vi "Run.vi"(8 "error in (no error)":errorcluster, 10 "OTP Cluster Out":T1, 11 "LCR-Measurement in":refnum<class "OTP_LCR_Meas.lvclass">) -> (0 "error out":errorcluster, 1 "Parameters":cluster{"Name":string, "Value":string}[](array[cluster]), 2 "Canceled":bool, 3 "LCR-Measurement out":refnum<class "OTP_LCR_Meas.lvclass">)   [LabVIEW 2020, in "OTP_LCR_Meas.lvclass"]
doc: "This is the main test vi. It is here that the test is implemented."
uses:
  OTP_LCR_Meas.lvclass
  C:/Sandbox/Git_Sandbox/WiSpry Test Framework source code (LV20)/WiSpry Test Framework/Measurements/Measurement.lvclass
  Controls/OTP_Cluster.ctl
  Controls/Run States.ctl
  Instruments/LCR Meter/Controls/Function.ctl
  Devices/Controls/Change setting mode enum.ctl
  Measurement.lvclass/Measurement.ctl
  XML Handler/Controls/Result Cluster.ctl
  Support VI/Update parameters (single).vi
  Support VI/Update parameters (array).vi
  Measurement.lvclass
  Instruments/LCR Meter/LCR Meter.lvclass
  Devices/Device.lvclass
  Devices/PIC-device/PIC-Device.lvclass
  XML Handler/XML Handler.lvclass
  Instruments/Power Supply/Power Supply.lvclass
  Instruments/Digital Multimeter/Digital Multimeter.lvclass
panel:
  out "Tab Control":enum32{"Page 1", "Page 2"}(tab)
  out "XY Graph":T2(graph)
  out "Waveform Chart":dbl[](graph)
  in  "Cancel Button":bool
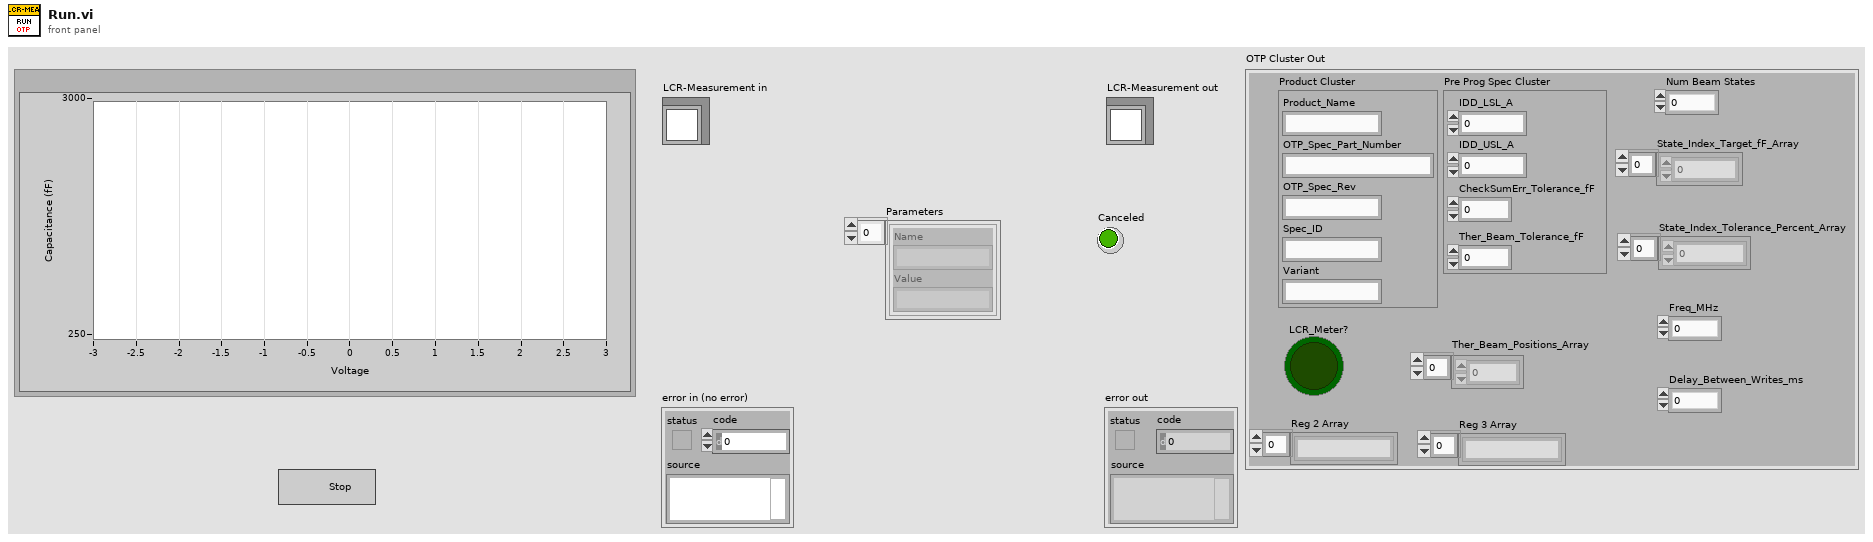
[diagram p1: front panel]
types:
  T1 = typedef "OTP_Cluster.ctl" = cluster{"Product Cluster":cluster{"Product_Name":string, "OTP_Spec_Part_Number":string, "OTP_Spec_Rev":string, "Spec_ID":string, "Variant":string}, "Pre Prog Spec Cluster":cluster{"IDD_LSL_A":dbl, "IDD_USL_A":dbl, "CheckSumErr_Tolerance_fF":dbl, "Ther_Beam_Tolerance_fF":dbl}, "LCR_Meter?":bool, "Reg 2 Array":string[], "Reg 3 Array":string[], "Num Beam States":i32, "State_Index_Target_fF_Array":dbl[], "State_Index_Tolerance_Percent_Array":dbl[], "Freq_MHz":dbl, "Delay_Between_Writes_ms":i32, "Ther_Beam_Positions_Array":i8[]}
  T2 = cluster{"Bias Voltages (V)":dbl[], "Capacitances (fF)":dbl[]}[]
  T3 = typedef "Measurement.lvclass/Run States.ctl" = enum16{"Init", "Set Device", "Read Environment", "Measure", "Done"}
  T4 = cluster{"Bias Voltages (V)":dbl[], "Capacitances (fF)":dbl[]}
  T5 = typedef "LCR Meter.lvclass/Function.ctl" = enum16{"Cp-D", "Cp-Q", "Cp-G", "Cp-Rp", "Cs-D", "Cs-Q", "Cs-Rs", "Lp-D", "Lp-Q", "Lp-G", "Lp-Rp", "Lp-Rdc", "Ls-D", "Ls-Q", "Ls-Rs", "Ls-Rdc", "R-X", "Z-thd", "Z-thr", "G-B", "Y-thd", "Y-thr", "Vdc-Idc"}
  T6 = typedef "PIC-Device.lvclass/Change setting mode enum.ctl" = enum16{"Init", "Next", "Reset"}
  T7 = typedef "XML Handler.lvclass/Result Cluster.ctl" = cluster{"Name":string, "Value":string}
  T8 = cluster{"Value":string, "Capacitance (fF)":string}
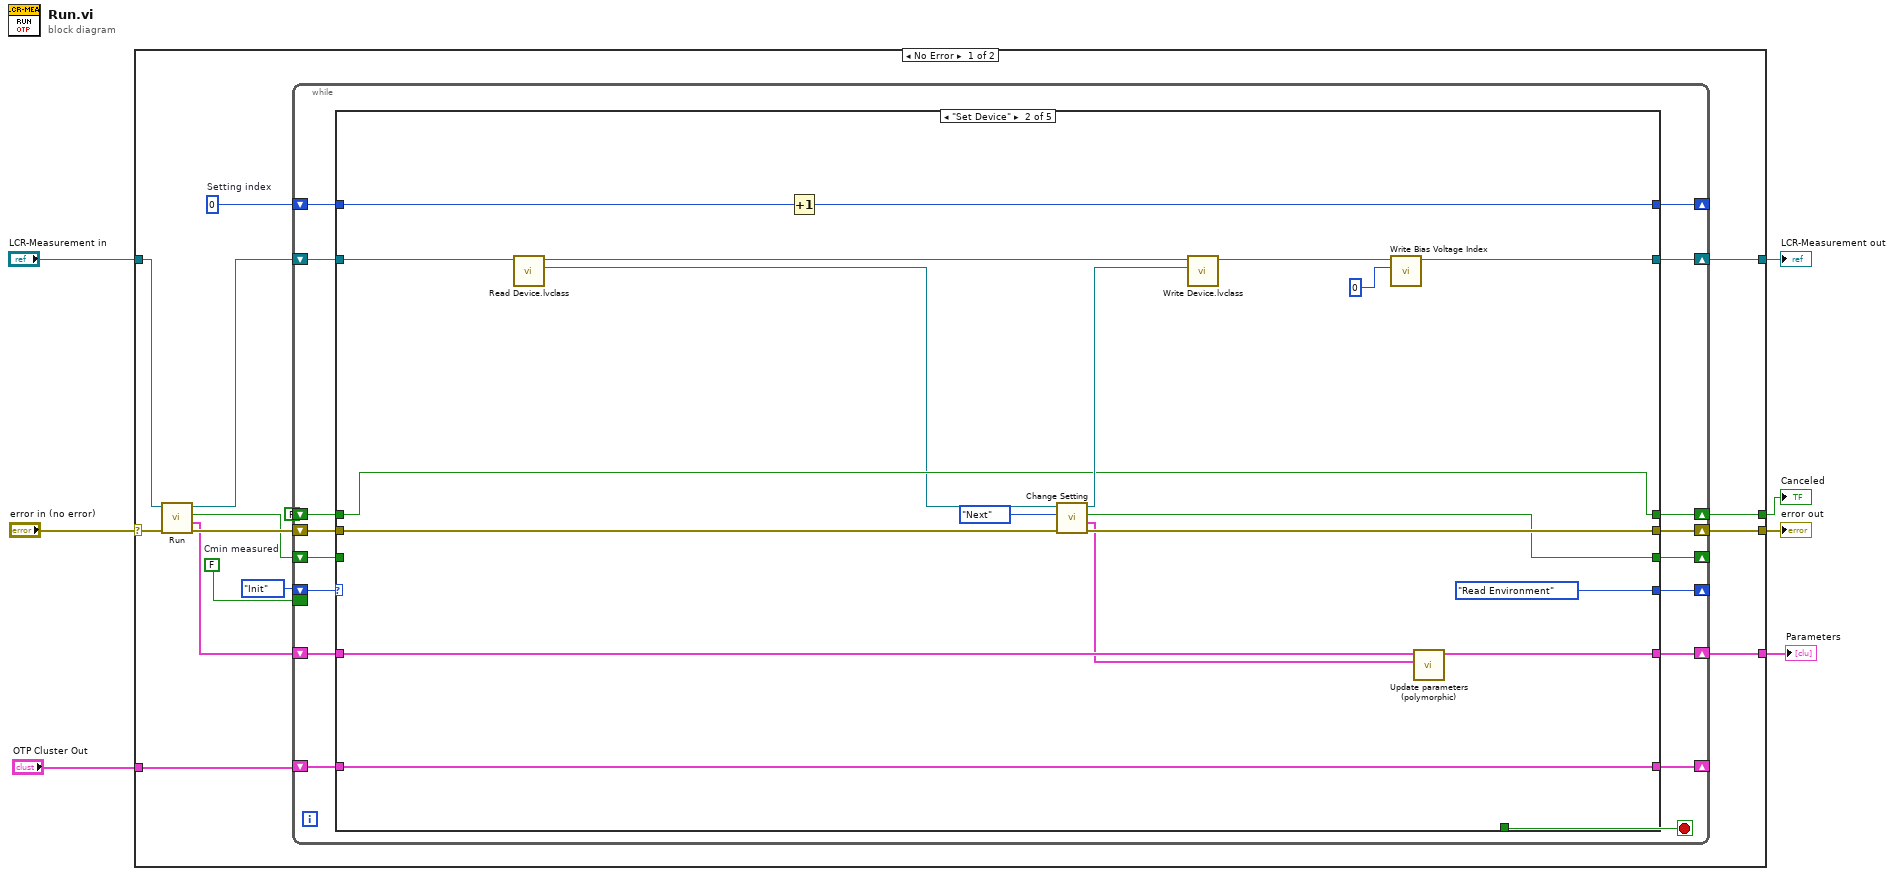
[diagram p0: block diagram]
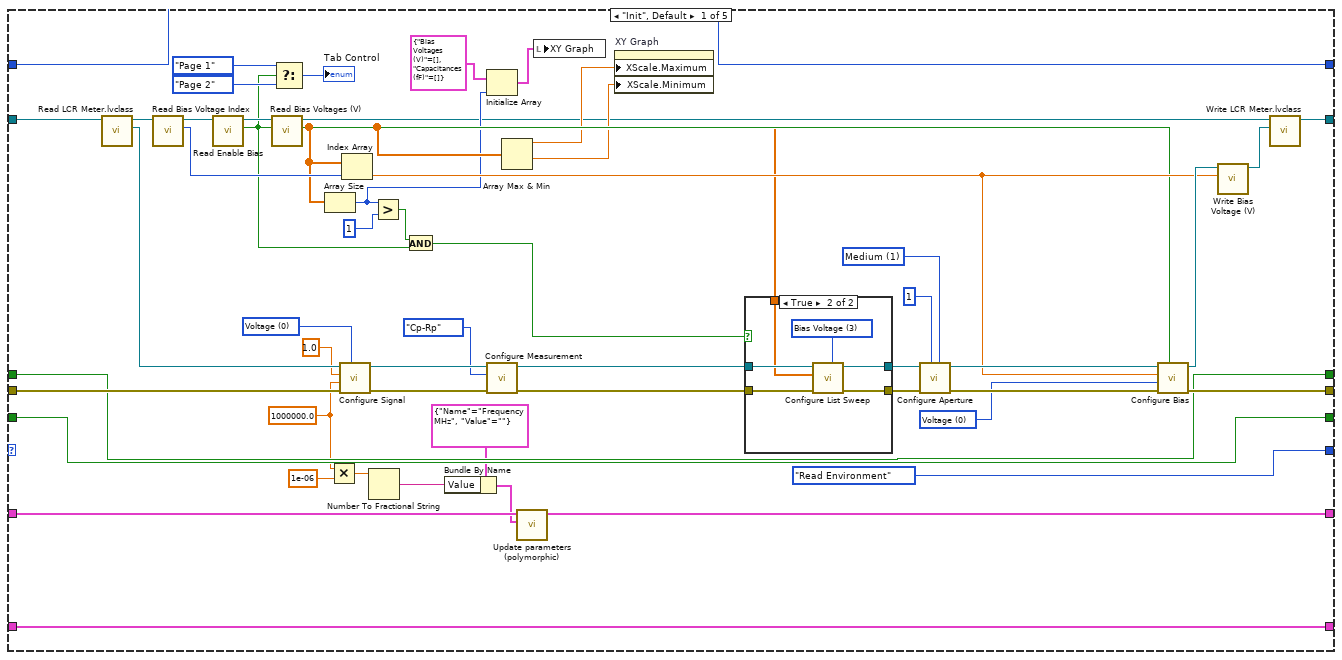
[diagram p2: hidden frame]
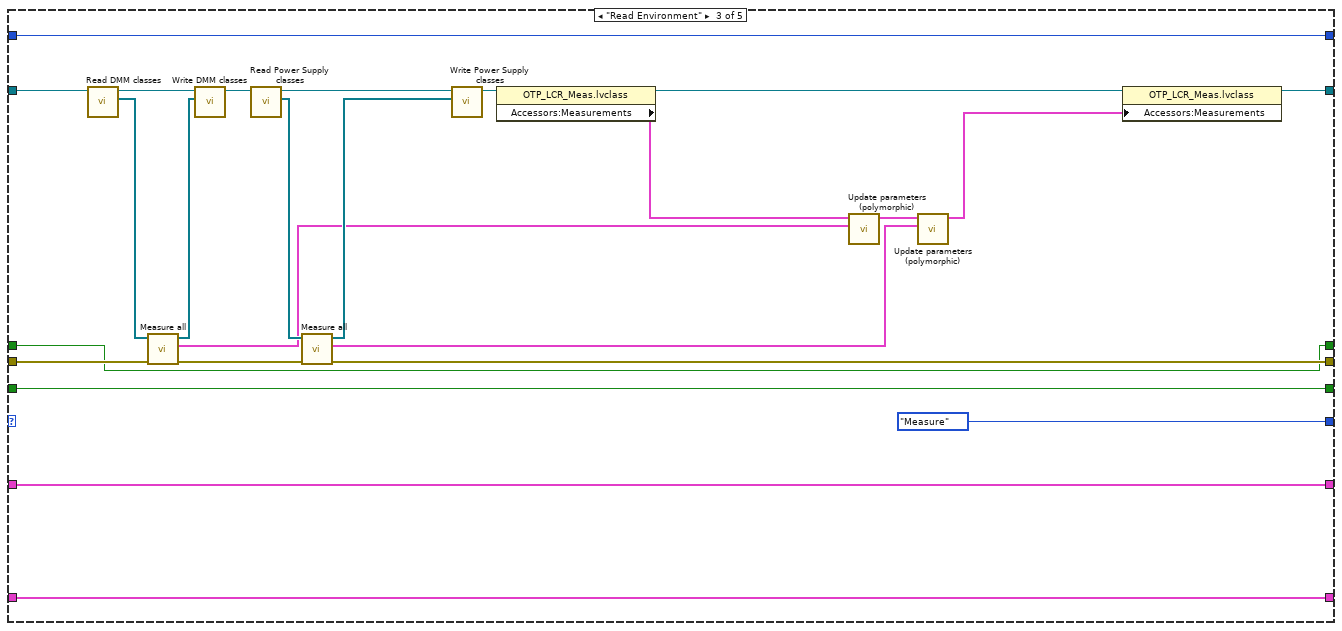
[diagram p4: hidden frame]
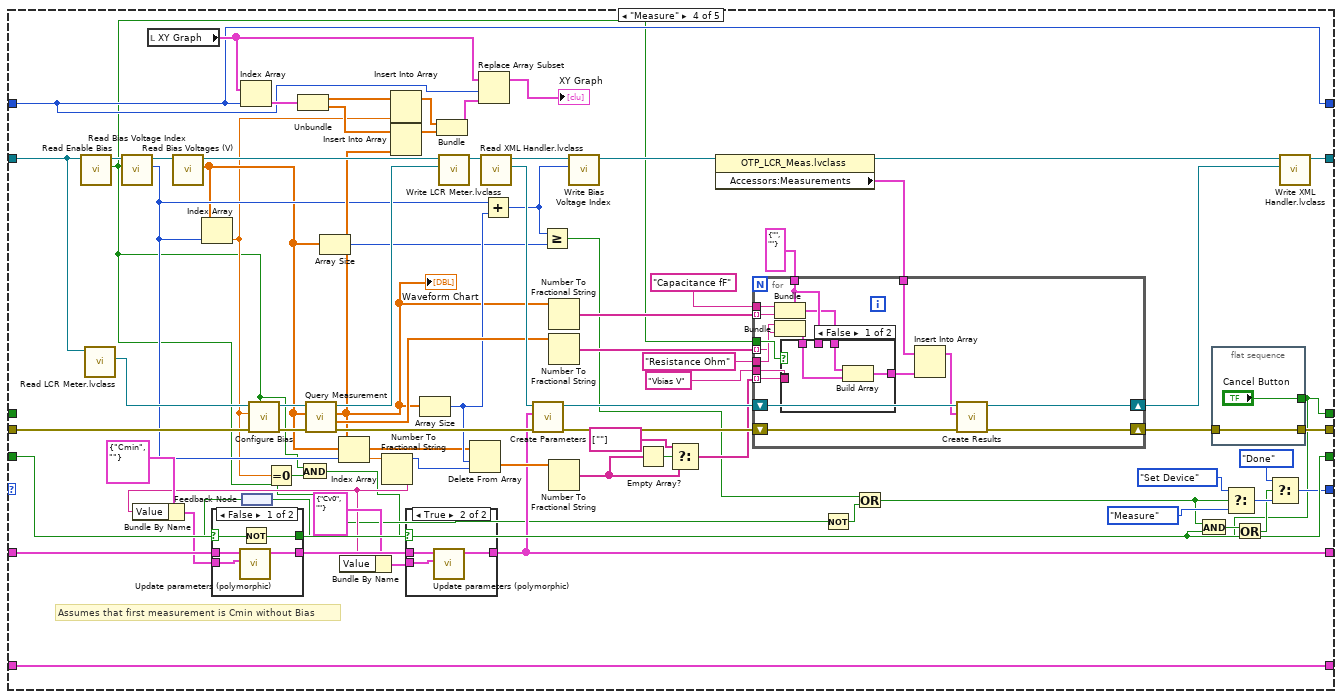
[diagram p5: hidden frame]
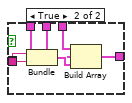
[diagram p8: hidden frame]
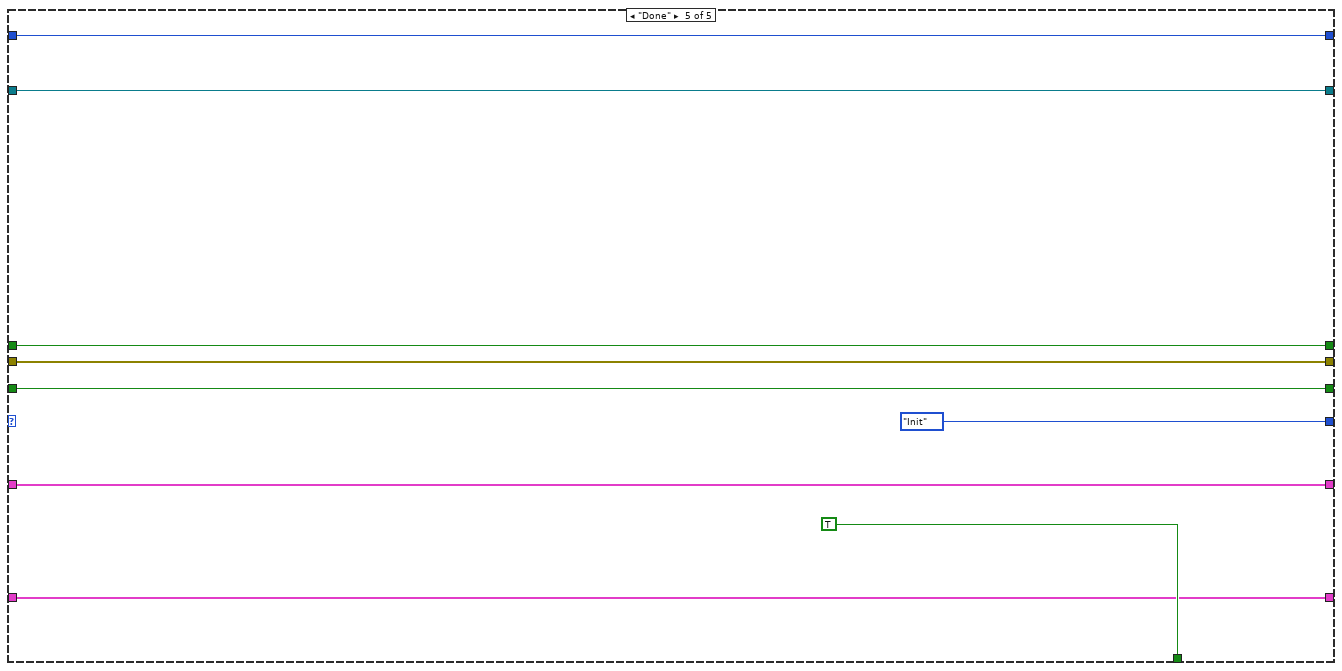
[diagram p9: hidden frame]
diagram:
  n1 = case shown="No Error" "error in (no error)" {
    selector: "error in (no error)" -> [w22 w272]
    tunnel: "LCR-Measurement in" -> [w21 w271]
    tunnel: [w19 w272] -> w6
    tunnel: [w17 w271] -> w5
    tunnel: [w16 _] -> w4
    tunnel: [w15 _] -> w3
    tunnel: "OTP Cluster Out" -> [w8 _]
    frame No Error {
      w10 = 0  # Setting index
      w11 = FALSE  # Cmin measured
      n2 = call-parent "Run.vi"("error in (no error)"=w22, "Measurements in"=w21) -> ("error out"=w20:errorcluster, "Parameters"=w12:cluster{"Name":string, "Value":string}[], "Canceled"=w14:bool, "Measurements out"=w18:refnum<class "OTP_LCR_Meas.lvclass">)  [unwired: 6 in]
      n3 = while {
        shift-right: [w38] -> w19
        shift-left: w20 -> [w39]
        shift-right: [w37] -> w17
        shift-left: w18 -> [w36]
        shift-right: [w34] -> _
        shift-left: Run_States."Init" ("Run states") -> [w25]
        shift-right: [w32] -> w15
        shift-left: w12 -> [w33]
        shift-right: [w31] -> _
        shift-left: w14 -> [w30]
        shift-right: [w28] -> w16
        shift-left: FALSE ("Cancel Button") -> [w29]
        border: w11 -> [_]
        shift-right: [w26] -> _
        shift-left: w10 -> [w27]
        shift-right: [w23] -> _
        shift-left: w8 -> [w24]
        stop <- w35 stop-if-true
        n4 = case shown="\"Set Device\"" w25 {
          tunnel: w39 -> [w84 w118 w136 w194 w270]
          tunnel: [w83 w117 w132 w183 w270] -> w38
          tunnel: [w81 w108 w127 w214 w269] -> w37
          tunnel: w36 -> [w82 w103 w143 w200 w269]
          tunnel: [_ _ _ _ TRUE] -> w35
          tunnel: [Run_States."Read Environment" ("Run states") Run_States."Read Environment" ("Run states") Run_States."Measure" ("Run states") w217 Run_States."Init" ("Run states")] -> w34
          tunnel: [w57 w109 w128 w181 w264] -> w28
          tunnel: w33 -> [w56 w114 w126 w177 w265]
          tunnel: [w55 w112 w126 w154 w265] -> w32
          tunnel: [w58 w110 w142 w219 w266] -> w31
          tunnel: w30 -> [w58 _ w142 w219 w266]
          tunnel: w29 -> [w57 w109 w128 _ w264]
          tunnel: w27 -> [w42 w105 w121 w162 w263]
          tunnel: [w42 w104 w121 w162 w263] -> w26
          tunnel: w24 -> [w40 w102 w120 w145 w262]
          tunnel: [w40 w102 w120 w145 w262] -> w23
          frame "Init", Default {
            w67 = u16 0 items=["Voltage", "Current"] ("DC Bias Type (0: Voltage)")
            w75 = u16 1 items=["Short", "Medium", "Long"] ("Measurement Time (1: Medium)")
            w53 = 1000000.0 ("Signal Frequency (1000 Hz)")
            w79 = u16 0 items=["Voltage", "Current"] ("Signal Type (0: Voltage)")
            n5 = call-dynamic "Read LCR Meter.lvclass.vi"("LCR-Measurement in"=w82) -> ("LCR Meter.lvclass"=w80:refnum<class "LCR Meter.lvclass">, "LCR-Measurement out"=w71:refnum<class "OTP_LCR_Meas.lvclass">)  [unwired: 9 in]
            n6 = call-dynamic "Read Bias Voltage Index.vi"("LCR-Measurement in"=w71) -> ("Bias Voltage Index"=w69:i32, "LCR-Measurement out"=w70:refnum<class "OTP_LCR_Meas.lvclass">)  [unwired: 9 in]
            n7 = call-dynamic "Read Enable Bias.vi"("LCR-Measurement in"=w70) -> ("Enable Bias"=w60:bool, "LCR-Measurement out"=w72:refnum<class "OTP_LCR_Meas.lvclass">)  [unwired: 9 in]
            n8 = call-dynamic "Read Bias Voltages (V).vi"("LCR-Measurement in"=w72) -> ("Bias Voltages (V)"=w48:dbl[], "LCR-Measurement out"=w41:refnum<class "OTP_LCR_Meas.lvclass">)  [unwired: 9 in]
            n9 = Select(t=enum32{"Page 1", "Page 2"}."Page 1" ("Tab Control"), s=w60, f=enum32{"Page 1", "Page 2"}."Page 2" ("Tab Control")) -> (s? t:f=→"Tab Control":enum32{"Page 1", "Page 2"})
            n10 = Array Size(array=w48) -> (size(s)=w44:i32)
            n11 = Multiply(x=w53, y=1e-06) -> (x*y=w51:dbl)
            n12 = call-dynamic "Configure Signal.vi"("Signal Type (0: Voltage)"=w79, "error in (no error)"=w84, "Signal Frequency (1 MHz)"=w53, "Signal Level (1.0 V)"=1.0, "LCR Meter in"=w80) -> ("error out"=w91:errorcluster, "LCR Meter out"=w92:refnum<class "LCR Meter.lvclass">)  [unwired: 5 in]
            n13 = Index Array(array=w48, index=w69) -> (element=w68:dbl)
            n14 = Number To Fractional String(number=w51) -> (F-format string=w50:string)  [unwired: 3 in]
            n15 = Greater?(x=w44, y=1) -> (0:w64:bool)
            n16 = And(x=w64, y=w60) -> (x .and. y?=w66:bool)
            n17 = Bundle By Name(cluster=cluster{"Name":string, "Value":string} {"Name"="Frequency MHz", "Value"=""} ("New Parameter"), "Value"=w50) -> (w49:cluster{"Name":string, "Value":string})
            n18 = Initialize Array(T4 {"Bias Voltages (V)"=[], "Capacitances (fF)"=[]} ("XY Graph"), w44) -> (w43:T2)
            n19 = call-dynamic "Configure Measurement.vi"("error in (no error)"=w91, "Function (0: Cp-D)"=Function."Cp-Rp", "LCR Meter in"=w92) -> ("error out"=w89:errorcluster, "LCR Meter out"=w90:refnum<class "LCR Meter.lvclass">)  [unwired: 7 in]
            n20 = Array Max & Min(array=w48) -> (max value=w47:dbl, min value=w46:dbl)  [unwired: 2 out]
            n21 = call-poly "Update parameters (polymorphic).vi"("New Parameter"=w49, "Parameters"=w56) -> ("Parameters Out"=w55:cluster{"Name":string, "Value":string}[])  [unwired: 9 in]
            n22 = local write "XY Graph"(w43) -> ()
            n23 = property on="XY Graph" class="XYGraph (strict)"("XScale.Maximum"=w47, "XScale.Minimum"=w46) -> ()  [unwired: 2 in, 2 out]
            n24 = case shown="True" w66 {
              tunnel: w90 -> [w94 w100]
              tunnel: w89 -> [w93 w99]
              tunnel: [w94 w98] -> w88
              tunnel: [w93 w97] -> w87
              tunnel: w48 -> [_ w96]
              frame False {
              }
              frame True {
                w95 = u16 3 items=["Frequency", "Voltage", "Current", "Bias Voltage", "Bias Current", "DC Source Voltage"] ("Sweep Function A (0: Frequency)")
                n25 = call-dynamic "Configure List Sweep.vi"("Sweep Function A (0: Frequency)"=w95, "error in (no error)"=w99, "Sweep Point Array"=w96, "LCR Meter in"=w100) -> ("error out"=w97:errorcluster, "LCR Meter out"=w98:refnum<class "LCR Meter.lvclass">)  [unwired: 6 in]
              }
            }
            n26 = call-dynamic "Configure Aperture.vi"("Measurement Time (1: Medium)"=w75, "Averaging Factor (1)"=1, "error in (no error)"=w87, "LCR Meter in"=w88) -> ("error out"=w85:errorcluster, "LCR Meter out"=w86:refnum<class "LCR Meter.lvclass">)  [unwired: 6 in]
            n27 = call-dynamic "Configure Bias.vi"("DC Bias State (F:Disable)"=w60, "error in (no error)"=w85, "DC Bias Type (0: Voltage)"=w67, "DC Bias Level (0.0 V)"=w68, "LCR Meter in"=w86) -> ("error out"=w83:errorcluster, "LCR Meter out"=w73:refnum<class "LCR Meter.lvclass">)  [unwired: 5 in]
            n28 = call-dynamic "Write Bias Voltage (V).vi"("Bias Voltage (V)"=w68, "LCR Meter in"=w73) -> ("LCR Meter out"=w74:refnum<class "LCR Meter.lvclass">)  [unwired: 9 in]
            n29 = call-dynamic "Write LCR Meter.lvclass.vi"("LCR Meter.lvclass"=w74, "LCR-Measurement in"=w41) -> ("LCR-Measurement out"=w81:refnum<class "OTP_LCR_Meas.lvclass">)  [unwired: 9 in]
          }
          frame "Set Device" {
            n30 = call "Read Device.lvclass.vi"("Measurements in"=w103) -> ("Device.lvclass"=w101:refnum<class "Device.lvclass">, "Measurements out"=w116:refnum<class "OTP_LCR_Meas.lvclass">)  [unwired: 9 in]
            n31 = Increment(x=w105) -> (x+1=w104:i32)
            n32 = call-dynamic "Change Setting.vi"("error in (no error)"=w118, "Change setting mode"=Change_setting_mode_enum."Next", "Device in"=w101) -> ("error out"=w117:errorcluster, "Changes"=w113:cluster{"Name":string, "Value":string}[], "Last setting"=w110:bool, "Device out"=w115:refnum<class "Device.lvclass">)  [unwired: 5 in]
            n33 = call "Write Device.lvclass.vi"("Device.lvclass"=w115, "Measurements in"=w116) -> ("Measurements out"=w107:refnum<class "OTP_LCR_Meas.lvclass">)  [unwired: 9 in]
            n34 = call-dynamic "Write Bias Voltage Index.vi"("Bias Voltage Index"=0, "LCR-Measurement in"=w107) -> ("LCR-Measurement out"=w108:refnum<class "OTP_LCR_Meas.lvclass">)  [unwired: 9 in]
            n35 = call-poly "Update parameters (polymorphic).vi"("New Parameters"=w113, "Parameters"=w114) -> ("Parameters Out"=w112:cluster{"Name":string, "Value":string}[])  [unwired: 9 in]
          }
          frame "Read Environment" {
            n36 = call-dynamic "Read DMM classes.vi"("Measurements in"=w143) -> ("DMM classes"=w133:refnum<class "Digital Multimeter.lvclass">[], "Measurements out"=w144:refnum<class "OTP_LCR_Meas.lvclass">)  [unwired: 9 in]
            n37 = call "Measure all.vi"("error in (no error)"=w136, "Digital Multimeters in"=w133) -> ("error out"=w135:errorcluster, "Measurements"=w131:T7[], "Digital Multimeters out"=w134:refnum<class "Digital Multimeter.lvclass">[])  [unwired: 5 in, 2 out]
            n38 = call-dynamic "Write DMM classes.vi"("DMM classes"=w134, "Measurements in"=w144) -> ("Measurements out"=w140:refnum<class "OTP_LCR_Meas.lvclass">)  [unwired: 9 in]
            n39 = call-dynamic "Read Power Supply classes.vi"("Measurements in"=w140) -> ("Power Supply classes"=w138:refnum<class "Power Supply.lvclass">[], "Measurements out"=w139:refnum<class "OTP_LCR_Meas.lvclass">)  [unwired: 9 in]
            n40 = call "Measure all.vi"("error in (no error)"=w135, "Power Supplies in"=w138) -> ("error out"=w132:errorcluster, "Measurements"=w129:T7[], "Power Supplies out"=w137:refnum<class "Power Supply.lvclass">[])  [unwired: 5 in, 2 out]
            n41 = call-dynamic "Write Power Supply classes.vi"("Power Supply classes"=w137, "Measurements in"=w139) -> ("Measurements out"=w124:refnum<class "OTP_LCR_Meas.lvclass">)  [unwired: 9 in]
            n42 = property class="OTP_LCR_Meas.lvclass"(reference=w124) -> (reference out=w123:refnum<class "OTP_LCR_Meas.lvclass">, "Accessors:Measurements"=w125:cluster{"Name":string, "Value":string}[])  [unwired: 1 in, 1 out]
            n43 = call-poly "Update parameters (polymorphic).vi"("New Parameters"=w131, "Parameters"=w125) -> ("Parameters Out"=w130:cluster{"Name":string, "Value":string}[])  [unwired: 9 in]
            n44 = call-poly "Update parameters (polymorphic).vi"("New Parameters"=w129, "Parameters"=w130) -> ("Parameters Out"=w122:cluster{"Name":string, "Value":string}[])  [unwired: 9 in]
            n45 = property class="OTP_LCR_Meas.lvclass"(reference=w123, "Accessors:Measurements"=w122) -> (reference out=w127:refnum<class "OTP_LCR_Meas.lvclass">)  [unwired: 1 in, 1 out]
          }
          frame "Measure" {
            # "Assumes that first measurement is Cmin without Bias"
            n46 = call-dynamic "Read Enable Bias.vi"("LCR-Measurement in"=w200) -> ("Enable Bias"=w148:bool, "LCR-Measurement out"=w178:refnum<class "OTP_LCR_Meas.lvclass">)  [unwired: 9 in]
            n47 = call-dynamic "Read LCR Meter.lvclass.vi"("LCR-Measurement in"=w200) -> ("LCR Meter.lvclass"=w191:refnum<class "LCR Meter.lvclass">)  [unwired: 9 in, 1 out]
            n48 = call-dynamic "Read Bias Voltage Index.vi"("LCR-Measurement in"=w178) -> ("Bias Voltage Index"=w161:i32, "LCR-Measurement out"=w180:refnum<class "OTP_LCR_Meas.lvclass">)  [unwired: 9 in]
            n49 = local read "XY Graph"() -> (w165:T2)
            n50 = call-dynamic "Read Bias Voltages (V).vi"("LCR-Measurement in"=w180) -> ("Bias Voltages (V)"=w158:dbl[], "LCR-Measurement out"=w179:refnum<class "OTP_LCR_Meas.lvclass">)  [unwired: 9 in]
            n51 = Index Array(array=w158, index=w161) -> (element=w150:dbl)
            n52 = Index Array(array=w165, index=w162) -> (element=w164:T4)
            n53 = feedback #1() -> (w176:bool)
            n54 = call-dynamic "Configure Bias.vi"("DC Bias State (F:Disable)"=w148, "error in (no error)"=w194, "DC Bias Level (0.0 V)"=w150, "LCR Meter in"=w191) -> ("error out"=w193:errorcluster, "LCR Meter out"=w192:refnum<class "LCR Meter.lvclass">)  [unwired: 6 in]
            n55 = Equal To 0?(x=w150) -> (x = 0?=w149:bool)
            n56 = Unbundle(w164) -> ("Bias Voltages (V)"=w171:dbl[], "Capacitances (fF)"=w170:dbl[])
            n57 = And(x=w148, y=w149) -> (x .and. y?=w147:bool)
            n58 = call-dynamic "Query Measurement.vi"("error in (no error)"=w193, "States"=w158, "LCR Meter in"=w192) -> ("error out"=w206:errorcluster, "Secondary results"=w197:dbl[], "Capacitances (fF)"=w169:dbl[], "LCR Meter out"=w210:refnum<class "LCR Meter.lvclass">)  [unwired: 5 in]
            "Waveform Chart" <- w169
            n59 = Array Size(array=w158) -> (size(s)=w157:i32)
            n60 = Index Array(array=w169) -> (element=w173:dbl)  [unwired: 1 in]
            n61 = Number To Fractional String(number=w173) -> (F-format string=w151:string)  [unwired: 3 in]
            n62 = Bundle By Name(cluster=cluster{"Name":string, "Value":string} {"Name"="Cmin", "Value"=""} ("Cluster"), "Value"=w151) -> (w172:cluster{"Name":string, "Value":string})
            n63 = case shown="False" w176 {
              selector: w176 -> [w228 w231]
              tunnel: w177 -> [w230 w232]
              tunnel: [w229 w232] -> w155
              tunnel: [w227 w231] -> w175
              tunnel: w172 -> [w226 _]
              frame False {
                n64 = call-poly "Update parameters (polymorphic).vi"("New Parameter"=w226, "Parameters"=w230) -> ("Parameters Out"=w229:cluster{"Name":string, "Value":string}[])  [unwired: 9 in]
                n65 = Not(x=w228) -> (.not. x?=w227:bool)
              }
              frame True {
              }
            }
            n66 = feedback-in #1(w175) -> ()
            n67 = Bundle By Name(cluster=cluster{"Name":string, "Value":string} {"Name"="Cv0", "Value"=""} ("Cluster"), "Value"=w151) -> (w152:cluster{"Name":string, "Value":string})
            n68 = Insert Into Array(array=w171, new element=w150) -> (w168:dbl[])  [unwired: 1 in]
            n69 = Insert Into Array(array=w170, new element=w169) -> (w167:dbl[])  [unwired: 1 in]
            n70 = case shown="True" w147 {
              tunnel: w155 -> [w222 w225]
              tunnel: [w222 w224] -> w154
              tunnel: w152 -> [_ w223]
              frame False {
              }
              frame True {
                n71 = call-poly "Update parameters (polymorphic).vi"("New Parameter"=w223, "Parameters"=w225) -> ("Parameters Out"=w224:cluster{"Name":string, "Value":string}[])  [unwired: 9 in]
              }
            }
            n72 = Array Size(array=w169) -> (size(s)=w190:i32)
            n73 = Bundle("Bias Voltages (V)"=w168, "Capacitances (fF)"=w167) -> (w163:T4)  [unwired: 1 in]
            n74 = call-dynamic "Write LCR Meter.lvclass.vi"("LCR Meter.lvclass"=w210, "LCR-Measurement in"=w179) -> ("LCR-Measurement out"=w209:refnum<class "OTP_LCR_Meas.lvclass">)  [unwired: 9 in]
            n75 = Delete From Array(array=w158, length=w190, index=w161) -> (deleted portion=w189:dbl[])  [unwired: 1 out]
            n76 = Replace Array Subset(array=w165, new element=w163, index=w162) -> (→"XY Graph":T2)
            n77 = call "Read XML Handler.lvclass.vi"("Measurements in"=w209) -> ("XML Handler.lvclass"=w212:refnum<class "XML Handler.lvclass">, "Measurements out"=w213:refnum<class "OTP_LCR_Meas.lvclass">)  [unwired: 9 in]
            n78 = Add(x=w161, y=w190) -> (x+y=w159:i32)
            n79 = call "Create Parameters.vi"("error in (no error)"=w206, "Parameters"=w154, "XML Handler in"=w212) -> ("error out"=w207:errorcluster, "XML Handler out"=w215:refnum<class "XML Handler.lvclass">)  [unwired: 7 in]
            n80 = Greater Or Equal?(x=w159, y=w157) -> (x >= y?=w156:bool)
            n81 = Number To Fractional String(number=w169) -> (F-format string=w203:string[])  [unwired: 3 in]
            n82 = Number To Fractional String(number=w197) -> (F-format string=w196:string[])  [unwired: 3 in]
            n83 = Number To Fractional String(number=w189) -> (F-format string=w160:string[])  [unwired: 3 in]
            n84 = call-dynamic "Write Bias Voltage Index.vi"("Bias Voltage Index"=w159, "LCR-Measurement in"=w213) -> ("LCR-Measurement out"=w188:refnum<class "OTP_LCR_Meas.lvclass">)  [unwired: 9 in]
            n85 = Empty Array?(array=w160) -> (empty?=w186:bool)
            n86 = Select(t=string[] [""], s=w186, f=w160) -> (s? t:f=w184:string[])
            n87 = property class="OTP_LCR_Meas.lvclass"(reference=w188) -> (reference out=w146:refnum<class "OTP_LCR_Meas.lvclass">, "Accessors:Measurements"=w187:cluster{"Name":string, "Value":string}[])  [unwired: 1 in, 1 out]
            n88 = for {
              shift-right: [w250] -> w211
              shift-left: w215 -> [w251]
              tunnel: T7 {"Name"="", "Value"=""} ("Result Cluster") -> [w249]
              shift-right: [w247] -> w182
              shift-left: w207 -> [w248]
              tunnel: "Capacitance fF" ("Value") -> [w246]
              tunnel: "Vbias V" ("Value") -> [w245]
              tunnel: w203 -> [w241] mode=indexing
              tunnel: w184 -> [w244] mode=indexing
              tunnel: w148 -> [w243]
              tunnel: w196 -> [w239] mode=indexing
              tunnel: "Resistance Ohm" ("Value") -> [w240]
              tunnel: w187 -> [w236]
              n89 = Bundle(cluster=w249, "Name"=w246, "Value"=w241) -> (w242:T7)
              n90 = Bundle("Value"=w240, "Capacitance (fF)"=w239) -> (w238:T8)  [unwired: 1 in]
              n91 = case shown="False" w243 {
                tunnel: w249 -> [_ w258]
                tunnel: w245 -> [_ w261]
                tunnel: w244 -> [_ w260]
                tunnel: w242 -> [w254 w257]
                tunnel: [w253 w256] -> w237
                tunnel: w238 -> [w252 w255]
                frame False {
                  n92 = Build Array(w254, w252) -> (w253:T7[])
                }
                frame True {
                  n93 = Bundle(cluster=w258, "Name"=w261, "Value"=w260) -> (w259:T7)
                  n94 = Build Array(w257, w255, w259) -> (w256:T7[])
                }
              }
              n95 = Insert Into Array(array=w236, new element=w237) -> (w235:cluster{"Name":string, "Value":string}[])  [unwired: 1 in]
              n96 = call "Create Results.vi"("error in (no error)"=w248, "Results"=w235, "XML Handler in"=w251) -> ("error out"=w247:errorcluster, "XML Handler out"=w250:refnum<class "XML Handler.lvclass">)  [unwired: 7 in]
            }
            n97 = Not(x=w148) -> (.not. x?=w198:bool)
            n98 = Or(x=w156, y=w198) -> (x .or. y?=w199:bool)
            n99 = And(x=w199, y=w219) -> (x .and. y?=w202:bool)
            n100 = flat-sequence {
              tunnel: [w234] -> w183
              tunnel: w182 -> [w234]
              tunnel: ["Cancel Button"] -> w181
              frame #0 {
              }
            }
            n101 = Select(t=Run_States."Set Device" ("Run states"), s=w199, f=Run_States."Measure" ("Run states")) -> (s? t:f=w218:T3)
            n102 = Or(x=w202, y=w181) -> (x .or. y?=w201:bool)
            n103 = Select(t=Run_States."Done" ("Run states"), s=w201, f=w218) -> (s? t:f=w217:T3)
            n104 = call "Write XML Handler.lvclass.vi"("XML Handler.lvclass"=w211, "Measurements in"=w146) -> ("Measurements out"=w214:refnum<class "OTP_LCR_Meas.lvclass">)  [unwired: 9 in]
          }
          frame "Done" {
          }
        }
      }
    }
    frame Error {
    }
  }
  "error out" <- w6
  "LCR-Measurement out" <- w5
  "Canceled" <- w4
  "Parameters" <- w3
